vi "Drive Base Immediate With Deadband.vi"(6 "Operation":T1, 7 "Description":string, 8 "Command Info In":T2, 9 "Deadband Value":dbl=0.01, 10 "Right Setpoint":dbl, 11 "Left Setpoint":dbl) -> (0 "Command Info Out":T2)   [LabVIEW 2019]
doc: "This template includes code for deadband comparision to avoid excessive command scheduling. It is particularly useful for joystick-driven commands.\n\nBe sure to right-click and select New from Template and save with a new command name."
uses:
  <vilib>/Rock Robotics/WPI/Framework/Command Status Info.ctl
  <vilib>/Rock Robotics/WPI/Framework/Completion Status.ctl
  <vilib>/Rock Robotics/WPI/Framework/Completion Notifier.ctl
  Implementation/Drive Base Operations.ctl
  Implementation/Drive Base Setpoints.ctl
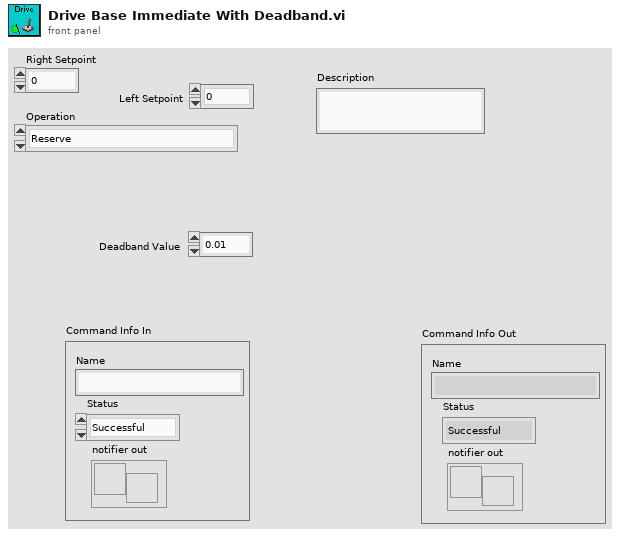
[diagram p1: front panel]
types:
  T1 = typedef "Drive Base Operations.ctl" = enum16{"Reserve", "Read Current", "Immediate", "Limelight"}
  T2 = typedef "Command Status Info.ctl" = cluster{"Name":string, "Status":T3, "notifier out":T4}
  T3 = typedef "Completion Status.ctl" = enum16{"Successful", "Aborted", "Incomplete"}
  T4 = typedef "Completion Notifier.ctl" = refnum<notifier>
  T5 = typedef "Drive Base Setpoints.ctl" = cluster{"Operation":T1, "Left Setpoint":dbl, "Duration":dbl, "Right Setpoint":dbl}
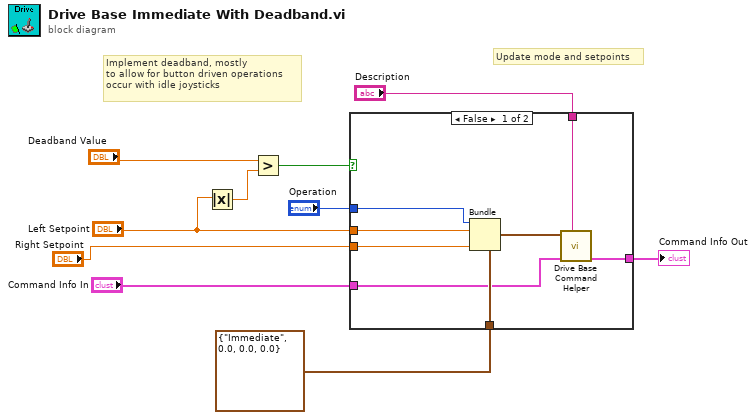
[diagram p0: block diagram]
diagram:
  # "Implement deadband, mostly\nto allow for button driven operations\noccur with idle joysticks"
  # "Update mode and setpoints"
  n1 = Absolute Value(x="Left Setpoint") -> (abs(x)=w9:dbl)
  n2 = Greater?(x="Deadband Value", y=w9) -> (0:w3:bool)
  n3 = case shown="False" w3 {
    tunnel: "Left Setpoint" -> [w18 _]
    tunnel: T5 {"Operation"=enum."Immediate", "Left Setpoint"=0.0, "Duration"=0.0, "Right Setpoint"=0.0} ("SubSystem Data") -> [w17 _]
    tunnel: [w16 w19] -> w8
    tunnel: "Command Info In" -> [w15 w19]
    tunnel: "Description" -> [w13 _]
    tunnel: "Right Setpoint" -> [w12 _]
    tunnel: "Operation" -> [w11 _]
    frame False {
      n4 = Bundle(cluster=w17, "Operation"=w11, "Left Setpoint"=w18, "Right Setpoint"=w12) -> (w14:T5)  [unwired: 1 in]
      n5 = call "Drive Base Command Helper.vi"("Description"=w13, "Command Info In"=w15, "SubSystem Data"=w14) -> ("Command Info Out"=w16:T2)  [unwired: 6 in, 2 out]
    }
    frame True {
    }
  }
  "Command Info Out" <- w8
